vi "PH_GetPowermeterInformation.panel.vi"(0 "object ref":refnum<vi>, 5 "error in (no error)":errorcluster) -> (19 "error out":errorcluster)   [LabVIEW 2014, in "PH_GetPowermeterInformation.lvlib"]
doc: "By this VI infoamation about cams is indicated.\n\n\"EXIT\" closes the front panel (GUI), while \"Delete Instance\" disconnects and removes the instance from the PCS.\n\n\nLicense Agreement for this software:\n\nCopyright (C)\nGesellschaft für Schwerionenforschung, GSI\nPlanckstr. 1\n64291 Darmstadt\nGermany\n\nContact: D.Beck@gsi.de \n\nThis program is free software; you can redistribute it and/or modify it under the terms of the GNU General Public License as published by the Free Software Foundation; either version 2 of the license, or (at your option) any later version.\n\nThis program is distributed in the hope that it will be useful, but WITHOUT ANYW ARRANTY; without even the implied warranty of MERCHANTABILITY or FITNESS FOR A PARTICULAR PURPOSE. See the GNU General License for more details (http://www.gnu.org).\n\nGesellschaft für Schwerionenforschung, GSI\nPlanckstr. 1, 64291 Darmstadt, Germany\nFor all questions and ideas contact: M.Richter@gsi.de, H.Brand@gsi.de or D.Beck@gsi.de.\nLast update: 18-DEC-2002"
uses:
  PH_GetPowermeterInformation.lvlib
  PH_Basics/PH_Common/PH_Common.lvlib
  PH_Basics/PH_GUI_Class/PH_GUI_Class.lvlib
panel:
  out "PCS Powermeter List":i32(listbox)
  in  "Save Information":bool
  in  "Get Information":bool
  in  "Delete":bool
  # "PCS"
  # "3.40"
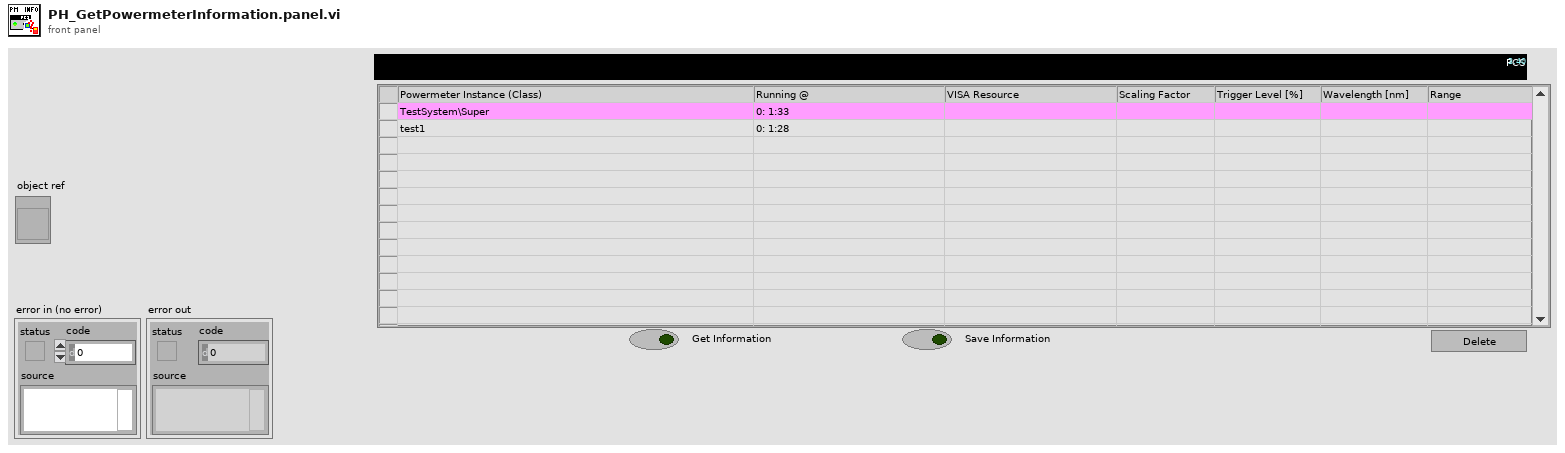
[diagram p1: front panel]
types:
  T1 = enum32{"Invalid", "Standard", "Closed", "Hidden", "Minimized", "Maximized"}
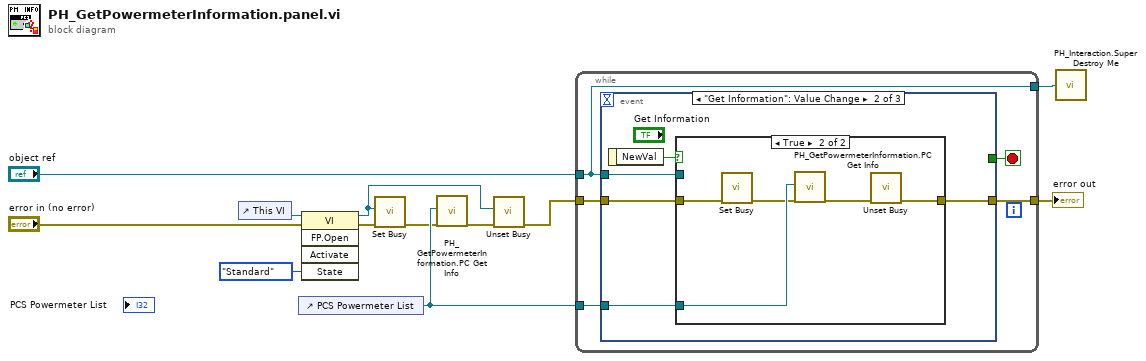
[diagram p0: block diagram]
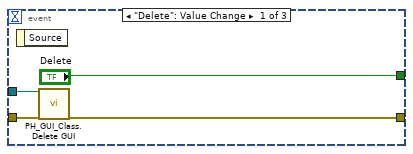
[diagram p2: hidden frame]
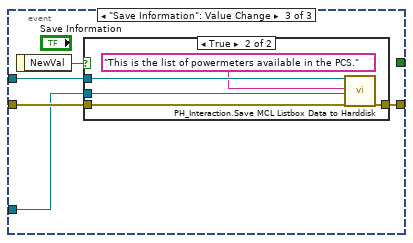
[diagram p4: hidden frame]
diagram:
  n1 = control-ref of="This VI"() -> (w7:refnum<vi>)
  n2 = control-ref of="PCS Powermeter List"() -> (w9:refnum<vi>)
  n3 = invoke class="VI" method="FP.Open"(reference=w7, error in="error in (no error)", "State"=T1."Standard") -> (reference out=w1:refnum<vi>, error out=w6:errorcluster)  [unwired: 2 in, 3 out]
  n4 = call <vilib>:"Set Busy.vi"("error in (no error)"=w6, "VI reference (current VI)"=w1) -> ("error out"=w4:errorcluster)  [unwired: 8 in, 1 out]
  n5 = call "PH_GetPowermeterInformation.PC Get Info.vi"("MCL Listbox GUI Ref"=w9, "error in"=w4) -> ("error out"=w3:errorcluster)  [unwired: 17 in]
  n6 = call <vilib>:"Unset Busy.vi"("error in (no error)"=w3, "VI reference (current VI)"=w1) -> ("error out"=w2:errorcluster)  [unwired: 9 in]
  n7 = while {
    tunnel: "object ref" -> [w16]
    tunnel: [w16] -> w12
    tunnel: w2 -> [w15]
    tunnel: [w14] -> w11
    tunnel: w9 -> [w13]
    stop <- w17 stop-if-true
    n8 = event shown="[1] \"Get Information\": Value Change" {
      selector: _ -> [_ _ _]
      dyn-events: _ -> [_ _ _]
      timeout: _ -> [_ _ _]
      tunnel: ["Delete" _ _] -> w17
      tunnel: w16 -> [w21 w24 w35]
      tunnel: w15 -> [w19 w26 w37]
      tunnel: [w18 w25 w36] -> w14
      tunnel: w13 -> [_ w22 w33]
      event "Delete": Value Change {
        n9 = event-data() -> ()  [unwired: 1 in, 1 out]
        n10 = call "PH_GUI_Class.Delete GUI.vi"("VI in"=w21, "error in (no error)"=w19) -> ("error out"=w18:errorcluster)  [unwired: 16 in, 1 out]
      }
      event "Get Information": Value Change {
        n11 = event-data() -> ("NewVal"=w23:bool)  [unwired: 1 in]
        n12 = case shown="True" w23 {
          tunnel: w26 -> [w27 w31]
          tunnel: [w27 w28] -> w25
          tunnel: w24 -> [_ _]
          tunnel: w22 -> [_ w32]
          frame False {
          }
          frame True {
            n13 = call <vilib>:"Set Busy.vi"("error in (no error)"=w31) -> ("error out"=w30:errorcluster)  [unwired: 9 in, 1 out]
            n14 = call "PH_GetPowermeterInformation.PC Get Info.vi"("MCL Listbox GUI Ref"=w32, "error in"=w30) -> ("error out"=w29:errorcluster)  [unwired: 17 in]
            n15 = call <vilib>:"Unset Busy.vi"("error in (no error)"=w29) -> ("error out"=w28:errorcluster)  [unwired: 10 in]
          }
        }
      }
      event "Save Information": Value Change {
        n16 = event-data() -> ("NewVal"=w34:bool)  [unwired: 1 in]
        n17 = case shown="True" w34 {
          tunnel: w37 -> [w38 w43]
          tunnel: [w38 w42] -> w36
          tunnel: w35 -> [_ w41]
          tunnel: w33 -> [_ w40]
          frame False {
          }
          frame True {
            n18 = call "PH_Interaction.Save MCL Listbox Data to Harddisk.vi"("VI in"=w41, "Headline"="This is the list of powermeters available in the PCS." ("string"), "MCL Listbox GUI Reference"=w40, "error in (no error)"=w43) -> ("error out"=w42:errorcluster)  [unwired: 14 in, 1 out]
          }
        }
      }
    }
  }
  "error out" <- w11
  n19 = call "PH_Interaction.Super Destroy Me.vi"("i ref out"=w12) -> ()
